vi "Acquire Scope data.vi"(8 "error in":errorcluster, 9 "Channels to read in":i32[](array[numeric]), 10 "input settings":T1={"LeCroy IP"="169.254.20.90", "Ch1"={"On/Off"=FALSE, "Bandwidth (Dropdown)"=0, "Vertical Range (V)"=5000.0, "Vertical Offset (V)"=0.0}, "Ch2"={"On/Off"=FALSE, "Bandwidth (Dropdown)"=0, "Vertical Range (V)"=0.2, "Vertical Offset (V)"=0.0}, "Ch3"={"On/Off"=TRUE, "Bandwidth (Dropdown)"=0, "Vertical Range (V)"=1.2, "Vertical Offset (V)"=0.0}, "Ch4"={"On/Off"=TRUE, "Bandwidth (Dropdown)"=0, "Vertical Range (V)"=0.2, "Vertical Offset (V)"=0.0}, "T axis"={"Time base (s/div)"=0.0002, "Time offset (s)"=0.0, "Max Sample Points"=0}, "Trig"={"Trigger mode"=2, "Trigger Slope"=0, "Trigger Source"=1, "Trigger Level (V)"=0.04}, "Timeout (ms)"=0.0} caption="Settings" {"Trig"."Trigger mode" items=["Auto", "Normal", "Single", "Single, auto trigger"]; "Trig"."Trigger Slope" items=["Rising", "Falling"]; "Trig"."Trigger Source" items=["Channel 1", "Channel 2", "Channel 3", "Channel 4", "External", "Power Line"]; "Trig"."Trigger Level (V)" format="%#_6p"; "T axis"."Max Sample Points" format="%.0p" items=["50"=50, "100"=100, "250"=250, "500"=500, "1000"=1000, "2500"=2500, "5K"=5000, "10K"=10000, "25K"=25000, "50K"=50000, "100K"=100000, "250K"=250000, "500K"=500000, "1M"=1000000, "2M"=2000000, "2.5M"=2500000, "5M"=5000000, "10M"=10000000, "25M"=25000000, "50M"=50000000, "100M"=100000000]; "T axis"."Time base (s/div)" format="%#_6p"; "Ch4"."Bandwidth (Dropdown)" items=["Full", "20MHZ", "25MHZ", "200MHZ", "250MHZ", "1GHZ", "3GHZ", "4GHZ"]; "Ch3"."Bandwidth (Dropdown)" items=["Full", "20MHZ", "25MHZ", "200MHZ", "250MHZ", "1GHZ", "3GHZ", "4GHZ"]; "Ch2"."Bandwidth (Dropdown)" items=["Full", "20MHZ", "25MHZ", "200MHZ", "250MHZ", "1GHZ", "3GHZ", "4GHZ"]; "Ch1"."Bandwidth (Dropdown)" items=["Full", "20MHZ", "25MHZ", "200MHZ", "250MHZ", "1GHZ", "3GHZ", "4GHZ"]}, 11 "VISA resource name in":refnum<visa-resource-name>) -> (0 "error out":errorcluster, 2 "output settings":T1={"LeCroy IP"="169.254.20.90", "Ch1"={"On/Off"=FALSE, "Bandwidth (Dropdown)"=0, "Vertical Range (V)"=5000.0, "Vertical Offset (V)"=0.0}, "Ch2"={"On/Off"=FALSE, "Bandwidth (Dropdown)"=0, "Vertical Range (V)"=0.2, "Vertical Offset (V)"=0.0}, "Ch3"={"On/Off"=TRUE, "Bandwidth (Dropdown)"=0, "Vertical Range (V)"=1.2, "Vertical Offset (V)"=0.0}, "Ch4"={"On/Off"=TRUE, "Bandwidth (Dropdown)"=0, "Vertical Range (V)"=0.2, "Vertical Offset (V)"=0.0}, "T axis"={"Time base (s/div)"=0.0002, "Time offset (s)"=0.0, "Max Sample Points"=0}, "Trig"={"Trigger mode"=2, "Trigger Slope"=0, "Trigger Source"=1, "Trigger Level (V)"=0.04}, "Timeout (ms)"=0.0} caption="Settings" {"Trig"."Trigger mode" items=["Auto", "Normal", "Single", "Single, auto trigger"]; "Trig"."Trigger Slope" items=["Rising", "Falling"]; "Trig"."Trigger Source" items=["Channel 1", "Channel 2", "Channel 3", "Channel 4", "External", "Power Line"]; "Trig"."Trigger Level (V)" format="%#_6p"; "T axis"."Max Sample Points" format="%.0p" items=["50"=50, "100"=100, "250"=250, "500"=500, "1000"=1000, "2500"=2500, "5K"=5000, "10K"=10000, "25K"=25000, "50K"=50000, "100K"=100000, "250K"=250000, "500K"=500000, "1M"=1000000, "2M"=2000000, "2.5M"=2500000, "5M"=5000000, "10M"=10000000, "25M"=25000000, "50M"=50000000, "100M"=100000000]; "T axis"."Time base (s/div)" format="%#_6p"; "Ch4"."Bandwidth (Dropdown)" items=["Full", "20MHZ", "25MHZ", "200MHZ", "250MHZ", "1GHZ", "3GHZ", "4GHZ"]; "Ch3"."Bandwidth (Dropdown)" items=["Full", "20MHZ", "25MHZ", "200MHZ", "250MHZ", "1GHZ", "3GHZ", "4GHZ"]; "Ch2"."Bandwidth (Dropdown)" items=["Full", "20MHZ", "25MHZ", "200MHZ", "250MHZ", "1GHZ", "3GHZ", "4GHZ"]; "Ch1"."Bandwidth (Dropdown)" items=["Full", "20MHZ", "25MHZ", "200MHZ", "250MHZ", "1GHZ", "3GHZ", "4GHZ"]}, 3 "VISA resource name out":refnum<visa-resource-name>, 5 "Waveform Data out":waveform(dbl)[](array[waveform]))   [LabVIEW 2013]
uses:
  Settings_TypeDef.ctl
  <instrlib>/LeCroy Wave Series/Public/Data/Read Multiple Waveforms.vi
  <instrlib>/LeCroy Wave Series/LeCroy Wave Series.lvlib
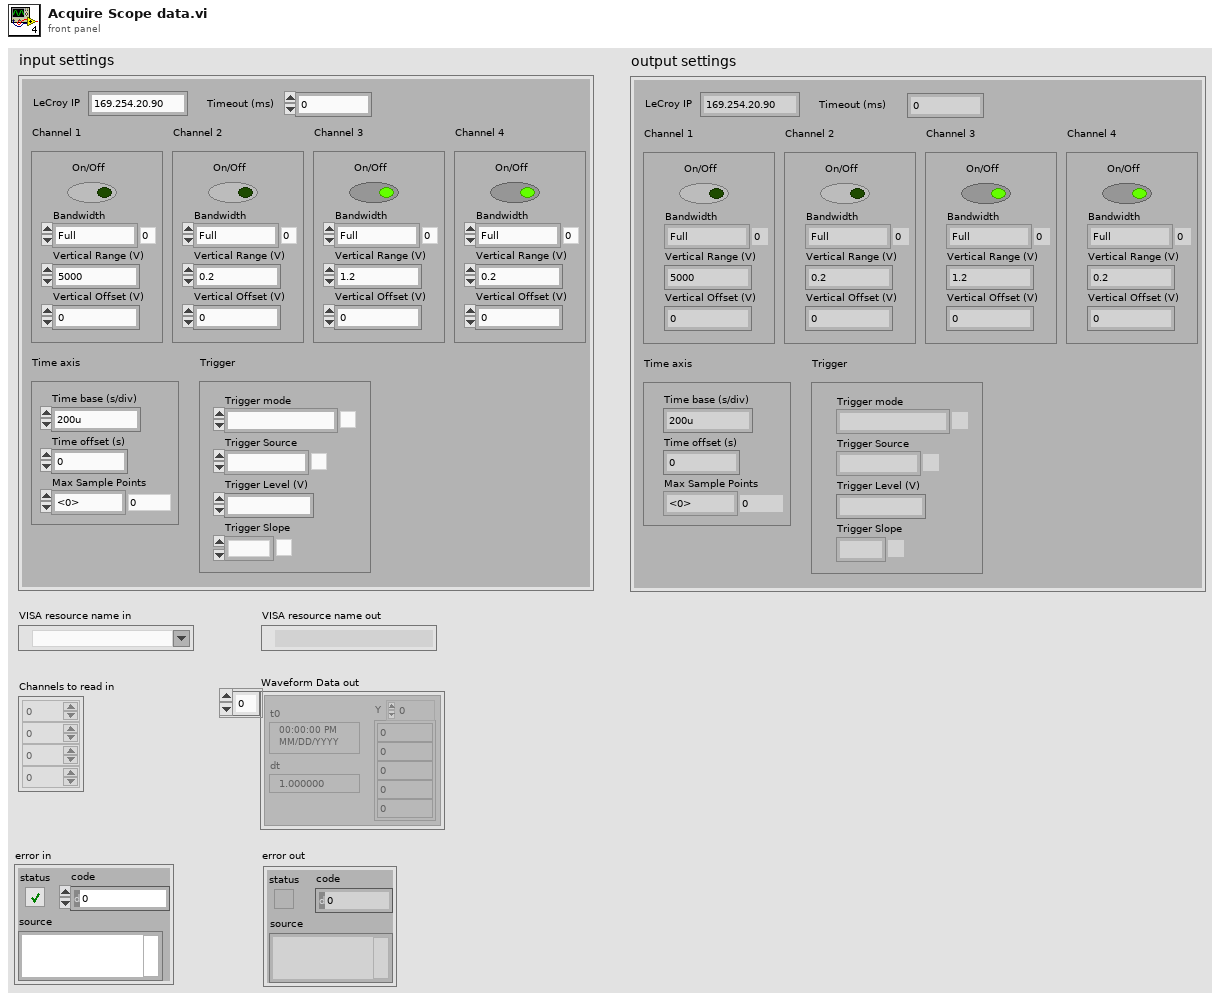
[diagram p1: front panel]
types:
  T1 = typedef "Settings_TypeDef.ctl" = cluster{"LeCroy IP":string, "Ch1":cluster{"On/Off":bool, "Bandwidth (Dropdown)":u16, "Vertical Range (V)":dbl, "Vertical Offset (V)":dbl}, "Ch2":cluster{"On/Off":bool, "Bandwidth (Dropdown)":u16, "Vertical Range (V)":dbl, "Vertical Offset (V)":dbl}, "Ch3":cluster{"On/Off":bool, "Bandwidth (Dropdown)":u16, "Vertical Range (V)":dbl, "Vertical Offset (V)":dbl}, "Ch4":cluster{"On/Off":bool, "Bandwidth (Dropdown)":u16, "Vertical Range (V)":dbl, "Vertical Offset (V)":dbl}, "T axis":cluster{"Time base (s/div)":dbl, "Time offset (s)":dbl, "Max Sample Points":i32}, "Trig":cluster{"Trigger mode":u16, "Trigger Slope":u16, "Trigger Source":u16, "Trigger Level (V)":dbl}, "Timeout (ms)":dbl}
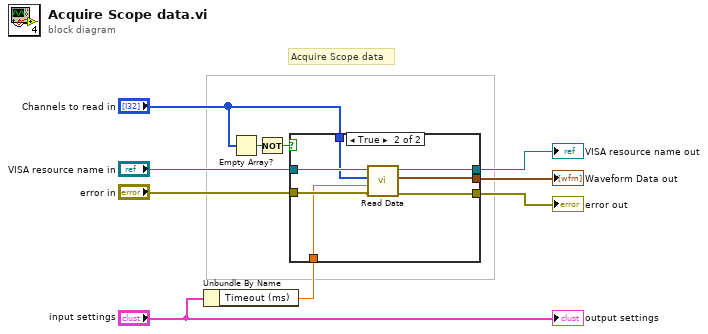
[diagram p0: block diagram]
diagram:
  # "Acquire Scope data"
  n1 = Unbundle By Name("input settings") -> ("Timeout (ms)"=w1:dbl)
  n2 = Empty Array?(array="Channels to read in") -> (empty?=w10:bool)
  n3 = Not(x=w10) -> (.not. x?=w9:bool)
  n4 = case shown="True" w9 {
    tunnel: [w12 w19] -> w3
    tunnel: "VISA resource name in" -> [w12 w18]
    tunnel: "error in" -> [w11 w17]
    tunnel: [w11 w16] -> w4
    tunnel: [_ w15] -> w7
    tunnel: "Channels to read in" -> [_ w14]
    tunnel: w1 -> [_ w13]
    frame False {
    }
    frame True {
      n5 = call-poly <instrlib>:"Read Data.vi"("error in (no error)"=w17, "Timeout (10000 ms)"=w13, "Channels"=w14, "VISA resource name"=w18) -> ("error out"=w16:errorcluster, "Waveform Data"=w15:waveform(dbl)[], "VISA resource name out"=w19:refnum<visa-resource-name>)  [unwired: 5 in]
    }
  }
  "Waveform Data out" <- w7
  "error out" <- w4
  "VISA resource name out" <- w3
  "output settings" <- "input settings"
